vi "PrepareAndSendSetROI.vi"(8 "error in (no error)":errorcluster, 9 "Clear ROI?(F)":bool=TRUE, 10 "ROI":T1, 11 "DisplayerUI in":refnum<class "DisplayerUI.lvclass">) -> (0 "error out":errorcluster, 3 "DisplayerUI out":refnum<class "DisplayerUI.lvclass">)   [LabVIEW 2020, in "Displayer.lvlib" / "DisplayerUI.lvlib" / "DisplayerUI.lvclass"]
uses:
  DisplayerUI.lvclass
  C:/Program Files/National Instruments/LabVIEW 2020/vi.lib/ActorFramework/Actor/Actor.lvclass
  <vilib>/ActorFramework/Actor/Actor.lvclass/Actor.ctl
  DisplayerUI.lvclass/DisplayerUI.ctl
  Displayer/Displayer Messages/SetROI Msg/SetROI Msg.lvclass/SetROI Msg.ctl
  <vilib>/ActorFramework/Message Enqueuer/Message Enqueuer.lvclass/Message Enqueuer.ctl
  <vilib>/ActorFramework/Message Enqueuer/Enqueue.vi
  Displayer/Displayer Messages/SetROI Msg/SetROI Msg.lvclass
  C:/Program Files/National Instruments/LabVIEW 2020/vi.lib/ActorFramework/Message/Message.lvclass
  <vilib>/ActorFramework/Message Priority Queue/Priority Enqueue.vi
  <vilib>/ActorFramework/Actor/Actor.lvclass
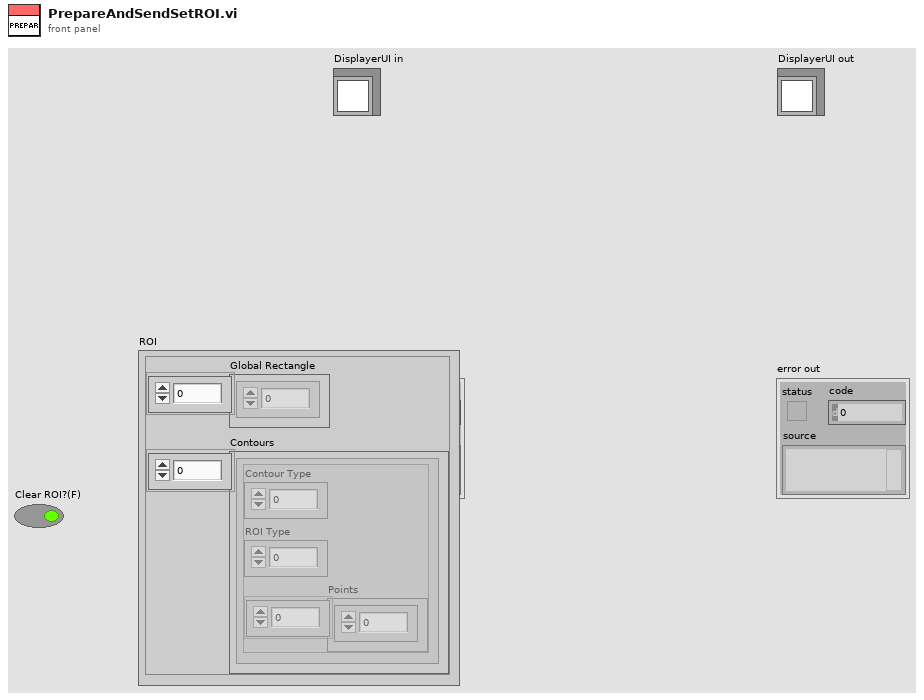
[diagram p1: front panel]
types:
  T1 = cluster{"Global Rectangle":i32[], "Contours":cluster{"Contour Type":u32, "ROI Type":u32, "Points":i32[]}[]}
  T2 = cluster{"x":dbl, "y":dbl, "width":dbl, "height":dbl}
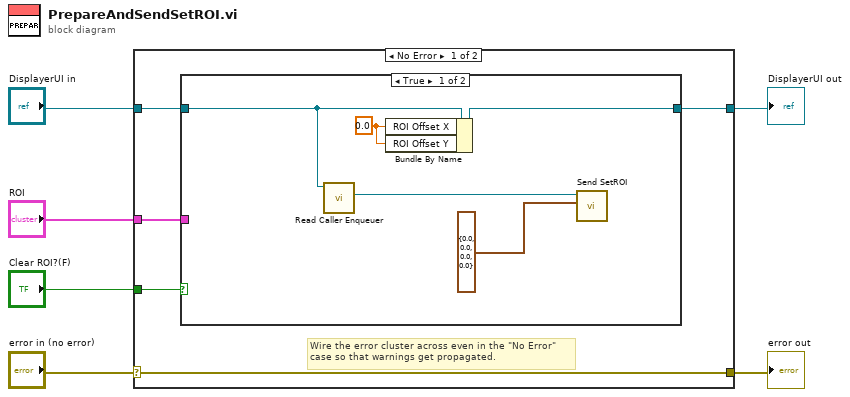
[diagram p0: block diagram]
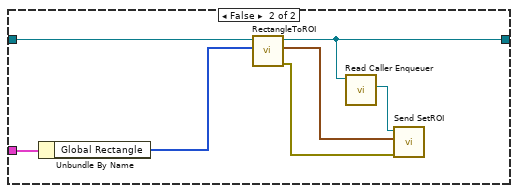
[diagram p2: hidden frame]
diagram:
  n1 = case shown="No Error" "error in (no error)" {
    selector: "error in (no error)" -> [w11 w25]
    tunnel: [w11 w25] -> w1
    tunnel: [w8 w24] -> w2
    tunnel: "DisplayerUI in" -> [w9 w24]
    tunnel: "ROI" -> [w10 _]
    tunnel: "Clear ROI?(F)" -> [w7 _]
    frame No Error {
      # "Wire the error cluster across even in the \"No Error\"\ncase so that warnings get propagated."
      n2 = case shown="True" w7 {
        tunnel: w10 -> [_ w23]
        tunnel: w9 -> [w14 w22]
        tunnel: [w16 w20] -> w8
        frame True {
          w15 = 0.0 ("ROI Offset X")
          n3 = call <vilib>:"Read Caller Enqueuer.vi"("Actor"=w14) -> ("Caller Enqueuer"=w13:refnum<class "Message Enqueuer.lvclass">)  [unwired: 10 in]
          n4 = Bundle By Name(cluster=w14, "ROI Offset X"=w15, "ROI Offset Y"=w15) -> (w16:refnum<class "DisplayerUI.lvclass">)
          n5 = call "Send SetROI.vi"("Setting.ROI"=T2 {"x"=0.0, "y"=0.0, "width"=0.0, "height"=0.0}, "Message Enqueuer"=w13) -> ()  [unwired: 8 in, 2 out]
        }
        frame False {
          n6 = Unbundle By Name(w23) -> ("Global Rectangle"=w21:i32[])
          n7 = call-dynamic "RectangleToROI.vi"("Global Rectangle in"=w21, "DisplayerUI in"=w22) -> ("error out"=w17:errorcluster, "Setting.ROI"=w18:T2, "DisplayerUI out"=w20:refnum<class "DisplayerUI.lvclass">)  [unwired: 7 in]
          n8 = call <vilib>:"Read Caller Enqueuer.vi"("Actor"=w20) -> ("Caller Enqueuer"=w19:refnum<class "Message Enqueuer.lvclass">)  [unwired: 10 in]
          n9 = call "Send SetROI.vi"("error in (no error)"=w17, "Setting.ROI"=w18, "Message Enqueuer"=w19) -> ()  [unwired: 7 in, 2 out]
        }
      }
    }
    frame Error {
    }
  }
  "error out" <- w1
  "DisplayerUI out" <- w2
